vi "Test - Draw Teapot.vi"() -> ()   [LabVIEW 2022 SP3, in "Raster.lvlib"] (continued)
"y"=79.69716, "z"=0.98665166}, "UV"={"u"=0.0, "v"=0.0}, "Colour"=12517256}, "Alpha"=0.0, "Alpha Blending Enabled"=FALSE, "Colour"=131841}, {"Vertex 1"={"Position"={"x"=284.21167, "y"=415.62677, "z"=0.9870124}, "UV"={"u"=0.0, "v"=0.0}, "Colour"=12517256}, "Vertex 2"={"Position"={"x"=286.22012, "y"=416.7535, "z"=0.987065}, "UV"={"u"=0.0, "v"=0.0}, "Colour"=12517256}, "Vertex 3"={"Position"={"x"=308.5938, "y"=420.3274, "z"=0.9866676}, "UV"={"u"=0.0, "v"=0.0}, "Colour"=12517256}, "Alpha"=0.0, "Alpha Blending Enabled"=FALSE, "Colour"=11463293}, {"Vertex 1"={"Position"={"x"=457.236, "y"=406.36896, "z"=0.98676956}, "UV"={"u"=0.0, "v"=0.0}, "Colour"=12517256}, "Vertex 2"={"Position"={"x"=455.76038, "y"=411.28638, "z"=0.98685414}, "UV"={"u"=0.0, "v"=0.0}, "Colour"=12517256}, "Vertex 3"={"Position"={"x"=479.31567, "y"=409.0878, "z"=0.98711485}, "UV"={"u"=0.0, "v"=0.0}, "Colour"=12517256}, "Alpha"=0.0, "Alpha Blending Enabled"=FALSE, "Colour"=11595134}, {"Vertex 1"={"Position"={"x"=218.37251, "y"=136.46829, "z"=0.98655325}, "UV"={"u"=0.0, "v"=0.0}, "Colour"=12517256}, "Vertex 2"={"Position"={"x"=228.17778, "y"=127.85439, "z"=0.98674196}, "UV"={"u"=0.0, "v"=0.0}, "Colour"=12517256}, "Vertex 3"={"Position"={"x"=214.19673, "y"=136.68369, "z"=0.9874245}, "UV"={"u"=0.0, "v"=0.0}, "Colour"=12517256}, "Alpha"=0.0, "Alpha Blending Enabled"=FALSE, "Colour"=131841}, {"Vertex 1"={"Position"={"x"=523.7792, "y"=100.105064, "z"=0.9868028}, "UV"={"u"=0.0, "v"=0.0}, "Colour"=12517256}, "Vertex 2"={"Position"={"x"=527.92816, "y"=103.53234, "z"=0.986694}, "UV"={"u"=0.0, "v"=0.0}, "Colour"=12517256}, "Vertex 3"={"Position"={"x"=546.8862, "y"=111.29832, "z"=0.9872219}, "UV"={"u"=0.0, "v"=0.0}, "Colour"=12517256}, "Alpha"=0.0, "Alpha Blending Enabled"=FALSE, "Colour"=131841}, {"Vertex 1"={"Position"={"x"=429.0421, "y"=412.70264, "z"=0.9866862}, "UV"={"u"=0.0, "v"=0.0}, "Colour"=12517256}, "Vertex 2"={"Position"={"x"=426.95547, "y"=415.24643, "z"=0.98692787}, "UV"={"u"=0.0, "v"=0.0}, "Colour"=12517256}, "Vertex 3"={"Position"={"x"=451.80063, "y"=413.90112, "z"=0.987081}, "UV"={"u"=0.0, "v"=0.0}, "Colour"=12517256}, "Alpha"=0.0, "Alpha Blending Enabled"=FALSE, "Colour"=11726719}, {"Vertex 1"={"Position"={"x"=488.21274, "y"=84.37186, "z"=0.98678565}, "UV"={"u"=0.0, "v"=0.0}, "Colour"=12517256}, "Vertex 2"={"Position"={"x"=480.10406, "y"=86.833496, "z"=0.9870857}, "UV"={"u"=0.0, "v"=0.0}, "Colour"=12517256}, "Vertex 3"={"Position"={"x"=456.3261, "y"=82.49355, "z"=0.9868217}, "UV"={"u"=0.0, "v"=0.0}, "Colour"=12517256}, "Alpha"=0.0, "Alpha Blending Enabled"=FALSE, "Colour"=131841}, {"Vertex 1"={"Position"={"x"=513.7799, "y"=416.7535, "z"=0.987065}, "UV"={"u"=0.0, "v"=0.0}, "Colour"=12517256}, "Vertex 2"={"Position"={"x"=515.7883, "y"=415.62677, "z"=0.9870124}, "UV"={"u"=0.0, "v"=0.0}, "Colour"=12517256}, "Vertex 3"={"Position"={"x"=493.06995, "y"=419.2306, "z"=0.986606}, "UV"={"u"=0.0, "v"=0.0}, "Colour"=12517256}, "Alpha"=0.0, "Alpha Blending Enabled"=FALSE, "Colour"=11463293}, {"Vertex 1"={"Position"={"x"=344.2396, "y"=411.28638, "z"=0.98685414}, "UV"={"u"=0.0, "v"=0.0}, "Colour"=12517256}, "Vertex 2"={"Position"={"x"=342.764, "y"=406.36896, "z"=0.98676956}, "UV"={"u"=0.0, "v"=0.0}, "Colour"=12517256}, "Vertex 3"={"Position"={"x"=318.62802, "y"=404.213, "z"=0.98703873}, "UV"={"u"=0.0, "v"=0.0}, "Colour"=12517256}, "Alpha"=0.0, "Alpha Blending Enabled"=FALSE, "Colour"=11595134}, {"Vertex 1"={"Position"={"x"=277.7324, "y"=405.7855, "z"=0.9868424}, "UV"={"u"=0.0, "v"=0.0}, "Colour"=12517256}, "Vertex 2"={"Position"={"x"=269.55508, "y"=385.5468, "z"=0.98662794}, "UV"={"u"=0.0, "v"=0.0}, "Colour"=12517256}, "Vertex 3"={"Position"={"x"=250.34036, "y"=382.10144, "z"=0.98716855}, "UV"={"u"=0.0, "v"=0.0}, "Colour"=12517256}, "Alpha"=0.0, "Alpha Blending Enabled"=FALSE, "Colour"=9881963}, {"Vertex 1"={"Position"={"x"=451.80063, "y"=413.90112, "z"=0.987081}, "UV"={"u"=0.0, "v"=0.0}, "Colour"=12517256}, "Vertex 2"={"Position"={"x"=455.76038, "y"=411.28638, "z"=0.98685414}, "UV"={"u"=0.0, "v"=0.0}, "Colour"=12517256}, "Vertex 3"={"Position"={"x"=429.0421, "y"=412.70264, "z"=0.9866862}, "UV"={"u"=0.0, "v"=0.0}, "Colour"=12517256}, "Alpha"=0.0, "Alpha Blending Enabled"=FALSE, "Colour"=11726719}, {"Vertex 1"={"Position"={"x"=425.18686, "y"=85.50133, "z"=0.9871326}, "UV"={"u"=0.0, "v"=0.0}, "Colour"=12517256}, "Vertex 2"={"Position"={"x"=429.3405, "y"=79.69716, "z"=0.98665166}, "UV"={"u"=0.0, "v"=0.0}, "Colour"=12517256}, "Vertex 3"={"Position"={"x"=456.3261, "y"=82.49355, "z"=0.9868217}, "UV"={"u"=0.0, "v"=0.0}, "Colour"=12517256}, "Alpha"=0.0, "Alpha Blending Enabled"=FALSE, "Colour"=131841}, {"Vertex 1"={"Position"={"x"=571.8222, "y"=127.85439, "z"=0.98674196}, "UV"={"u"=0.0, "v"=0.0}, "Colour"=12517256}, "Vertex 2"={"Position"={"x"=581.62744, "y"=136.46829, "z"=0.98655325}, "UV"={"u"=0.0, "v"=0.0}, "Colour"=12517256}, "Vertex 3"={"Position"={"x"=595.8332, "y"=145.30861, "z"=0.9872829}, "UV"={"u"=0.0, "v"=0.0}, "Colour"=12517256}, "Alpha"=0.0, "Alpha Blending Enabled"=FALSE, "Colour"=131841}, {"Vertex 1"={"Position"={"x"=282.04407, "y"=413.45215, "z"=0.9869555}, "UV"={"u"=0.0, "v"=0.0}, "Colour"=12517256}, "Vertex 2"={"Position"={"x"=284.21167, "y"=415.62677, "z"=0.9870124}, "UV"={"u"=0.0, "v"=0.0}, "Colour"=12517256}, "Vertex 3"={"Position"={"x"=306.93005, "y"=419.2306, "z"=0.986606}, "UV"={"u"=0.0, "v"=0.0}, "Colour"=12517256}, "Alpha"=0.0, "Alpha Blending Enabled"=FALSE, "Colour"=11594878}, {"Vertex 1"={"Position"={"x"=549.6596, "y"=382.10144, "z"=0.98716855}, "UV"={"u"=0.0, "v"=0.0}, "Colour"=12517256}, "Vertex 2"={"Position"={"x"=558.7478, "y"=361.91916, "z"=0.9869936}, "UV"={"u"=0.0, "v"=0.0}, "Colour"=12517256}, "Vertex 3"={"Position"={"x"=538.7197, "y"=364.68237, "z"=0.986411}, "UV"={"u"=0.0, "v"=0.0}, "Colour"=12517256}, "Alpha"=0.0, "Alpha Blending Enabled"=FALSE, "Colour"=9816171}, {"Vertex 1"={"Position"={"x"=613.1543, "y"=168.46658, "z"=0.9870382}, "UV"={"u"=0.0, "v"=0.0}, "Colour"=12517256}, "Vertex 2"={"Position"={"x"=605.2505, "y"=155.83162, "z"=0.98714983}, "UV"={"u"=0.0, "v"=0.0}, "Colour"=12517256}, "Vertex 3"={"Position"={"x"=590.8862, "y"=147.17273, "z"=0.98637503}, "UV"={"u"=0.0, "v"=0.0}, "Colour"=12517256}, "Alpha"=0.0, "Alpha Blending Enabled"=FALSE, "Colour"=790537}, {"Vertex 1"={"Position"={"x"=188.08968, "y"=258.6834, "z"=0.9870558}, "UV"={"u"=0.0, "v"=0.0}, "Colour"=12517256}, "Vertex 2"={"Position"={"x"=194.1895, "y"=278.80545, "z"=0.98714197}, "UV"={"u"=0.0, "v"=0.0}, "Colour"=12517256}, "Vertex 3"={"Position"={"x"=208.56157, "y"=277.5288, "z"=0.9863644}, "UV"={"u"=0.0, "v"=0.0}, "Colour"=12517256}, "Alpha"=0.0, "Alpha Blending Enabled"=FALSE, "Colour"=8037207}, {"Vertex 1"={"Position"={"x"=562.28735, "y"=121.01229, "z"=0.9869255}, "UV"={"u"=0.0, "v"=0.0}, "Colour"=12517256}, "Vertex 2"={"Position"={"x"=553.7546, "y"=115.60594, "z"=0.98708975}, "UV"={"u"=0.0, "v"=0.0}, "Colour"=12517256}, "Vertex 3"={"Position"={"x"=534.1681, "y"=107.647095, "z"=0.9865303}, "UV"={"u"=0.0, "v"=0.0}, "Colour"=12517256}, "Alpha"=0.0, "Alpha Blending Enabled"=FALSE, "Colour"=131841}, {"Vertex 1"={"Position"={"x"=306.38147, "y"=83.88072, "z"=0.98658574}, "UV"={"u"=0.0, "v"=0.0}, "Colour"=12517256}, "Vertex 2"={"Position"={"x"=311.7873, "y"=84.37186, "z"=0.98678565}, "UV"={"u"=0.0, "v"=0.0}, "Colour"=12517256}, "Vertex 3"={"Position"={"x"=290.0812, "y"=90.55896, "z"=0.9871663}, "UV"={"u"=0.0, "v"=0.0}, "Colour"=12517256}, "Alpha"=0.0, "Alpha Blending Enabled"=FALSE, "Colour"=131841}, {"Vertex 1"={"Position"={"x"=584.2917, "y"=298.96686, "z"=0.98650193}, "UV"={"u"=0.0, "v"=0.0}, "Colour"=12517256}, "Vertex 2"={"Position"={"x"=576.293, "y"=320.26297, "z"=0.98665595}, "UV"={"u"=0.0, "v"=0.0}, "Colour"=12517256}, "Vertex 3"={"Position"={"x"=590.3839, "y"=319.19806, "z"=0.9873598}, "UV"={"u"=0.0, "v"=0.0}, "Colour"=12517256}, "Alpha"=0.0, "Alpha Blending Enabled"=FALSE, "Colour"=8564573}, {"Vertex 1"={"Position"={"x"=515.7883, "y"=415.62677, "z"=0.9870124}, "UV"={"u"=0.0, "v"=0.0}, "Colour"=12517256}, "Vertex 2"={"Position"={"x"=517.956, "y"=413.45215, "z"=0.9869555}, "UV"={"u"=0.0, "v"=0.0}, "Colour"=12517256}, "Vertex 3"={"Position"={"x"=494.86752, "y"=417.05643, "z"=0.9865395}, "UV"={"u"=0.0, "v"=0.0}, "Colour"=12517256}, "Alpha"=0.0, "Alpha Blending Enabled"=FALSE, "Colour"=11594878}, {"Vertex 1"={"Position"={"x"=491.4062, "y"=420.3274, "z"=0.9866676}, "UV"={"u"=0.0, "v"=0.0}, "Colour"=12517256}, "Vertex 2"={"Position"={"x"=489.97534, "y"=420.3969, "z"=0.9867205}, "UV"={"u"=0.0, "v"=0.0}, "Colour"=12517256}, "Vertex 3"={"Position"={"x"=512.05084, "y"=416.87537, "z"=0.9871104}, "UV"={"u"=0.0, "v"=0.0}, "Colour"=12517256}, "Alpha"=0.0, "Alpha Blending Enabled"=FALSE, "Colour"=10343280}, {"Vertex 1"={"Position"={"x"=370.9579, "y"=412.70264, "z"=0.9866862}, "UV"={"u"=0.0, "v"=0.0}, "Colour"=12517256}, "Vertex 2"={"Position"={"x"=373.04453, "y"=415.24643, "z"=0.98692787}, "UV"={"u"=0.0, "v"=0.0}, "Colour"=12517256}, "Vertex 3"={"Position"={"x"=400.0, "y"=415.71765, "z"=0.98687416}, "UV"={"u"=0.0, "v"=0.0}, "Colour"=12517256}, "Alpha"=0.0, "Alpha Blending Enabled"=FALSE, "Colour"=11792768}, {"Vertex 1"={"Position"={"x"=520.2092, "y"=91.74848, "z"=0.9868964}, "UV"={"u"=0.0, "v"=0.0}, "Colour"=12517256}, "Vertex 2"={"Position"={"x"=516.44995, "y"=90.450294, "z"=0.986995}, "UV"={"u"=0.0, "v"=0.0}, "Colour"=12517256}, "Vertex 3"={"Position"={"x"=493.61853, "y"=83.88072, "z"=0.98658574}, "UV"={"u"=0.0, "v"=0.0}, "Colour"=12517256}, "Alpha"=0.0, "Alpha Blending Enabled"=FALSE, "Colour"=131841}, {"Vertex 1"={"Position"={"x"=373.04453, "y"=415.24643, "z"=0.98692787}, "UV"={"u"=0.0, "v"=0.0}, "Colour"=12517256}, "Vertex 2"={"Position"={"x"=370.9579, "y"=412.70264, "z"=0.9866862}, "UV"={"u"=0.0, "v"=0.0}, "Colour"=12517256}, "Vertex 3"={"Position"={"x"=344.2396, "y"=411.28638, "z"=0.98685414}, "UV"={"u"=0.0, "v"=0.0}, "Colour"=12517256}, "Alpha"=0.0, "Alpha Blending Enabled"=FALSE, "Colour"=11726719}, {"Vertex 1"={"Position"={"x"=310.02466, "y"=420.3969, "z"=0.9867205}, "UV"={"u"=0.0, "v"=0.0}, "Colour"=12517256}, "Vertex 2"={"Position"={"x"=308.5938, "y"=420.3274, "z"=0.9866676}, "UV"={"u"=0.0, "v"=0.0}, "Colour"=12517256}, "Vertex 3"={"Position"={"x"=286.22012, "y"=416.7535, "z"=0.987065}, "UV"={"u"=0.0, "v"=0.0}, "Colour"=12517256}, "Alpha"=0.0, "Alpha Blending Enabled"=FALSE, "Colour"=10343280}, {"Vertex 1"={"Position"={"x"=265.8319, "y"=107.647095, "z"=0.9865303}, "UV"={"u"=0.0, "v"=0.0}, "Colour"=12517256}, "Vertex 2"={"Position"={"x"=272.07184, "y"=103.53234, "z"=0.986694}, "UV"={"u"=0.0, "v"=0.0}, "Colour"=12517256}, "Vertex 3"={"Position"={"x"=253.11374, "y"=111.29832, "z"=0.9872219}, "UV"={"u"=0.0, "v"=0.0}, "Colour"=12517256}, "Alpha"=0.0, "Alpha Blending Enabled"=FALSE, "Colour"=131841}, {"Vertex 1"={"Position"={"x"=605.8105, "y"=278.80545, "z"=0.98714197}, "UV"={"u"=0.0, "v"=0.0}, "Colour"=12517256}, "Vertex 2"={"Position"={"x"=611.91034, "y"=258.6834, "z"=0.9870558}, "UV"={"u"=0.0, "v"=0.0}, "Colour"=12517256}, "Vertex 3"={"Position"={"x"=597.4648, "y"=256.11636, "z"=0.98624843}, "UV"={"u"=0.0, "v"=0.0}, "Colour"=12517256}, "Alpha"=0.0, "Alpha Blending Enabled"=FALSE, "Colour"=8037207}, {"Vertex 1"={"Position"={"x"=400.0, "y"=413.19934, "z"=0.98662734}, "UV"={"u"=0.0, "v"=0.0}, "Colour"=12517256}, "Vertex 2"={"Position"={"x"=400.0, "y"=415.71765, "z"=0.98687416}, "UV"={"u"=0.0, "v"=0.0}, "Colour"=12517256}, "Vertex 3"={"Position"={"x"=426.95547, "y"=415.24643, "z"=0.98692787}, "UV"={"u"=0.0, "v"=0.0}, "Colour"=12517256}, "Alpha"=0.0, "Alpha Blending Enabled"=FALSE, "Colour"=11792768}, {"Vertex 1"={"Position"={"x"=194.7495, "y"=155.83162, "z"=0.98714983}, "UV"={"u"=0.0, "v"=0.0}, "Colour"=12517256}, "Vertex 2"={"Position"={"x"=186.84569, "y"=168.46658, "z"=0.9870382}, "UV"={"u"=0.0, "v"=0.0}, "Colour"=12517256}, "Vertex 3"={"Position"={"x"=201.30348, "y"=160.24332, "z"=0.9862247}, "UV"={"u"=0.0, "v"=0.0}, "Colour"=12517256}, "Alpha"=0.0, "Alpha Blending Enabled"=FALSE, "Colour"=790537}, {"Vertex 1"={"Position"={"x"=223.70695, "y"=320.26297, "z"=0.98665595}, "UV"={"u"=0.0, "v"=0.0}, "Colour"=12517256}, "Vertex 2"={"Position"={"x"=215.7083, "y"=298.96686, "z"=0.98650193}, "UV"={"u"=0.0, "v"=0.0}, "Colour"=12517256}, "Vertex 3"={"Position"={"x"=201.45174, "y"=299.0235, "z"=0.9872445}, "UV"={"u"=0.0, "v"=0.0}, "Colour"=12517256}, "Alpha"=0.0, "Alpha Blending Enabled"=FALSE, "Colour"=8564573}, {"Vertex 1"={"Position"={"x"=337.8442, "y"=79.5276, "z"=0.98648775}, "UV"={"u"=0.0, "v"=0.0}, "Colour"=12517256}, "Vertex 2"={"Position"={"x"=343.6739, "y"=82.49355, "z"=0.9868217}, "UV"={"u"=0.0, "v"=0.0}, "Colour"=12517256}, "Vertex 3"={"Position"={"x"=319.8959, "y"=86.833496, "z"=0.9870857}, "UV"={"u"=0.0, "v"=0.0}, "Colour"=12517256}, "Alpha"=0.0, "Alpha Blending Enabled"=FALSE, "Colour"=131841}, {"Vertex 1"={"Position"={"x"=279.84146, "y"=410.18558, "z"=0.9868977}, "UV"={"u"=0.0, "v"=0.0}, "Colour"=12517256}, "Vertex 2"={"Position"={"x"=282.04407, "y"=413.45215, "z"=0.9869555}, "UV"={"u"=0.0, "v"=0.0}, "Colour"=12517256}, "Vertex 3"={"Position"={"x"=305.13248, "y"=417.05643, "z"=0.9865395}, "UV"={"u"=0.0, "v"=0.0}, "Colour"=12517256}, "Alpha"=0.0, "Alpha Blending Enabled"=FALSE, "Colour"=11331451}, {"Vertex 1"={"Position"={"x"=374.81314, "y"=85.50133, "z"=0.9871326}, "UV"={"u"=0.0, "v"=0.0}, "Colour"=12517256}, "Vertex 2"={"Position"={"x"=370.6595, "y"=79.69716, "z"=0.98665166}, "UV"={"u"=0.0, "v"=0.0}, "Colour"=12517256}, "Vertex 3"={"Position"={"x"=400.0, "y"=78.71635, "z"=0.986592}, "UV"={"u"=0.0, "v"=0.0}, "Colour"=12517256}, "Alpha"=0.0, "Alpha Blending Enabled"=FALSE, "Colour"=131841}, {"Vertex 1"={"Position"={"x"=488.21274, "y"=84.37186, "z"=0.98678565}, "UV"={"u"=0.0, "v"=0.0}, "Colour"=12517256}, "Vertex 2"={"Position"={"x"=493.61853, "y"=83.88072, "z"=0.98658574}, "UV"={"u"=0.0, "v"=0.0}, "Colour"=12517256}, "Vertex 3"={"Position"={"x"=516.44995, "y"=90.450294, "z"=0.986995}, "UV"={"u"=0.0, "v"=0.0}, "Colour"=12517256}, "Alpha"=0.0, "Alpha Blending Enabled"=FALSE, "Colour"=131841}, {"Vertex 1"={"Position"={"x"=283.55002, "y"=90.450294, "z"=0.986995}, "UV"={"u"=0.0, "v"=0.0}, "Colour"=12517256}, "Vertex 2"={"Position"={"x"=279.79077, "y"=91.74848, "z"=0.9868964}, "UV"={"u"=0.0, "v"=0.0}, "Colour"=12517256}, "Vertex 3"={"Position"={"x"=303.26147, "y"=85.00194, "z"=0.9864703}, "UV"={"u"=0.0, "v"=0.0}, "Colour"=12517256}, "Alpha"=0.0, "Alpha Blending Enabled"=FALSE, "Colour"=131841}, {"Vertex 1"={"Position"={"x"=319.8959, "y"=86.833496, "z"=0.9870857}, "UV"={"u"=0.0, "v"=0.0}, "Colour"=12517256}, "Vertex 2"={"Position"={"x"=311.7873, "y"=84.37186, "z"=0.98678565}, "UV"={"u"=0.0, "v"=0.0}, "Colour"=12517256}, "Vertex 3"={"Position"={"x"=337.8442, "y"=79.5276, "z"=0.98648775}, "UV"={"u"=0.0, "v"=0.0}, "Colour"=12517256}, "Alpha"=0.0, "Alpha Blending Enabled"=FALSE, "Colour"=131841}, {"Vertex 1"={"Position"={"x"=246.24544, "y"=115.60594, "z"=0.98708975}, "UV"={"u"=0.0, "v"=0.0}, "Colour"=12517256}, "Vertex 2"={"Position"={"x"=237.71262, "y"=121.01229, "z"=0.9869255}, "UV"={"u"=0.0, "v"=0.0}, "Colour"=12517256}, "Vertex 3"={"Position"={"x"=258.046, "y"=112.83853, "z"=0.98632616}, "UV"={"u"=0.0, "v"=0.0}, "Colour"=12517256}, "Alpha"=0.0, "Alpha Blending Enabled"=FALSE, "Colour"=131841}, {"Vertex 1"={"Position"={"x"=493.06995, "y"=419.2306, "z"=0.986606}, "UV"={"u"=0.0, "v"=0.0}, "Colour"=12517256}, "Vertex 2"={"Position"={"x"=491.4062, "y"=420.3274, "z"=0.9866676}, "UV"={"u"=0.0, "v"=0.0}, "Colour"=12517256}, "Vertex 3"={"Position"={"x"=513.7799, "y"=416.7535, "z"=0.987065}, "UV"={"u"=0.0, "v"=0.0}, "Colour"=12517256}, "Alpha"=0.0, "Alpha Blending Enabled"=FALSE, "Colour"=11463293}, {"Vertex 1"={"Position"={"x"=400.0, "y"=84.68199, "z"=0.98708326}, "UV"={"u"=0.0, "v"=0.0}, "Colour"=12517256}, "Vertex 2"={"Position"={"x"=400.0, "y"=78.71635, "z"=0.986592}, "UV"={"u"=0.0, "v"=0.0}, "Colour"=12517256}, "Vertex 3"={"Position"={"x"=429.3405, "y"=79.69716, "z"=0.98665166}, "UV"={"u"=0.0, "v"=0.0}, "Colour"=12517256}, "Alpha"=0.0, "Alpha Blending Enabled"=FALSE, "Colour"=131841}, {"Vertex 1"={"Position"={"x"=517.956, "y"=413.45215, "z"=0.9869555}, "UV"={"u"=0.0, "v"=0.0}, "Colour"=12517256}, "Vertex 2"={"Position"={"x"=520.1585, "y"=410.18558, "z"=0.9868977}, "UV"={"u"=0.0, "v"=0.0}, "Colour"=12517256}, "Vertex 3"={"Position"={"x"=496.69638, "y"=413.75363, "z"=0.9864719}, "UV"={"u"=0.0, "v"=0.0}, "Colour"=12517256}, "Alpha"=0.0, "Alpha Blending Enabled"=FALSE, "Colour"=11331451}, {"Vertex 1"={"Position"={"x"=527.92816, "y"=103.53234, "z"=0.986694}, "UV"={"u"=0.0, "v"=0.0}, "Colour"=12517256}, "Vertex 2"={"Position"={"x"=534.1681, "y"=107.647095, "z"=0.9865303}, "UV"={"u"=0.0, "v"=0.0}, "Colour"=12517256}, "Vertex 3"={"Position"={"x"=553.7546, "y"=115.60594, "z"=0.98708975}, "UV"={"u"=0.0, "v"=0.0}, "Colour"=12517256}, "Alpha"=0.0, "Alpha Blending Enabled"=FALSE, "Colour"=131841}, {"Vertex 1"={"Position"={"x"=342.764, "y"=406.36896, "z"=0.98676956}, "UV"={"u"=0.0, "v"=0.0}, "Colour"=12517256}, "Vertex 2"={"Position"={"x"=344.2396, "y"=411.28638, "z"=0.98685414}, "UV"={"u"=0.0, "v"=0.0}, "Colour"=12517256}, "Vertex 3"={"Position"={"x"=370.9579, "y"=412.70264, "z"=0.9866862}, "UV"={"u"=0.0, "v"=0.0}, "Colour"=12517256}, "Alpha"=0.0, "Alpha Blending Enabled"=FALSE, "Colour"=11990146}, {"Vertex 1"={"Position"={"x"=183.4162, "y"=238.81894, "z"=0.98698974}, "UV"={"u"=0.0, "v"=0.0}, "Colour"=12517256}, "Vertex 2"={"Position"={"x"=188.08968, "y"=258.6834, "z"=0.9870558}, "UV"={"u"=0.0, "v"=0.0}, "Colour"=12517256}, "Vertex 3"={"Position"={"x"=202.53506, "y"=256.11636, "z"=0.98624843}, "UV"={"u"=0.0, "v"=0.0}, "Colour"=12517256}, "Alpha"=0.0, "Alpha Blending Enabled"=FALSE, "Colour"=7576146}, {"Vertex 1"={"Position"={"x"=308.5938, "y"=420.3274, "z"=0.9866676}, "UV"={"u"=0.0, "v"=0.0}, "Colour"=12517256}, "Vertex 2"={"Position"={"x"=306.93005, "y"=419.2306, "z"=0.986606}, "UV"={"u"=0.0, "v"=0.0}, "Colour"=12517256}, "Vertex 3"={"Position"={"x"=284.21167, "y"=415.62677, "z"=0.9870124}, "UV"={"u"=0.0, "v"=0.0}, "Colour"=12517256}, "Alpha"=0.0, "Alpha Blending Enabled"=FALSE, "Colour"=11463293}, {"Vertex 1"={"Position"={"x"=426.95547, "y"=415.24643, "z"=0.98692787}, "UV"={"u"=0.0, "v"=0.0}, "Colour"=12517256}, "Vertex 2"={"Position"={"x"=429.0421, "y"=412.70264, "z"=0.9866862}, "UV"={"u"=0.0, "v"=0.0}, "Colour"=12517256}, "Vertex 3"={"Position"={"x"=400.0, "y"=413.19934, "z"=0.98662734}, "UV"={"u"=0.0, "v"=0.0}, "Colour"=12517256}, "Alpha"=0.0, "Alpha Blending Enabled"=FALSE, "Colour"=11792768}, {"Vertex 1"={"Position"={"x"=232.30115, "y"=341.28168, "z"=0.98682135}, "UV"={"u"=0.0, "v"=0.0}, "Colour"=12517256}, "Vertex 2"={"Position"={"x"=241.25218, "y"=361.91916, "z"=0.9869936}, "UV"={"u"=0.0, "v"=0.0}, "Colour"=12517256}, "Vertex 3"={"Position"={"x"=261.2803, "y"=364.68237, "z"=0.986411}, "UV"={"u"=0.0, "v"=0.0}, "Colour"=12517256}, "Alpha"=0.0, "Alpha Blending Enabled"=FALSE, "Colour"=9750378}, {"Vertex 1"={"Position"={"x"=618.5962, "y"=183.36784, "z"=0.98696136}, "UV"={"u"=0.0, "v"=0.0}, "Colour"=12517256}, "Vertex 2"={"Position"={"x"=613.1543, "y"=168.46658, "z"=0.9870382}, "UV"={"u"=0.0, "v"=0.0}, "Colour"=12517256}, "Vertex 3"={"Position"={"x"=598.69653, "y"=160.24332, "z"=0.9862247}, "UV"={"u"=0.0, "v"=0.0}, "Colour"=12517256}, "Alpha"=0.0, "Alpha Blending Enabled"=FALSE, "Colour"=2701085}, {"Vertex 1"={"Position"={"x"=455.76038, "y"=411.28638, "z"=0.98685414}, "UV"={"u"=0.0, "v"=0.0}, "Colour"=12517256}, "Vertex 2"={"Position"={"x"=457.236, "y"=406.36896, "z"=0.98676956}, "UV"={"u"=0.0, "v"=0.0}, "Colour"=12517256}, "Vertex 3"={"Position"={"x"=429.82074, "y"=407.75894, "z"=0.986596}, "UV"={"u"=0.0, "v"=0.0}, "Colour"=12517256}, "Alpha"=0.0, "Alpha Blending Enabled"=FALSE, "Colour"=11990146}, {"Vertex 1"={"Position"={"x"=521.88837, "y"=94.06487, "z"=0.98685235}, "UV"={"u"=0.0, "v"=0.0}, "Colour"=12517256}, "Vertex 2"={"Position"={"x"=520.2092, "y"=91.74848, "z"=0.9868964}, "UV"={"u"=0.0, "v"=0.0}, "Colour"=12517256}, "Vertex 3"={"Position"={"x"=496.73853, "y"=85.00194, "z"=0.9864703}, "UV"={"u"=0.0, "v"=0.0}, "Colour"=12517256}, "Alpha"=0.0, "Alpha Blending Enabled"=FALSE, "Colour"=988171}, {"Vertex 1"={"Position"={"x"=277.7324, "y"=405.7855, "z"=0.9868424}, "UV"={"u"=0.0, "v"=0.0}, "Colour"=12517256}, "Vertex 2"={"Position"={"x"=279.84146, "y"=410.18558, "z"=0.9868977}, "UV"={"u"=0.0, "v"=0.0}, "Colour"=12517256}, "Vertex 3"={"Position"={"x"=303.30362, "y"=413.75363, "z"=0.9864719}, "UV"={"u"=0.0, "v"=0.0}, "Colour"=12517256}, "Alpha"=0.0, "Alpha Blending Enabled"=FALSE, "Colour"=10870390}, {"Vertex 1"={"Position"={"x"=209.11378, "y"=147.17273, "z"=0.98637503}, "UV"={"u"=0.0, "v"=0.0}, "Colour"=12517256}, "Vertex 2"={"Position"={"x"=218.37251, "y"=136.46829, "z"=0.98655325}, "UV"={"u"=0.0, "v"=0.0}, "Colour"=12517256}, "Vertex 3"={"Position"={"x"=204.1668, "y"=145.30861, "z"=0.9872829}, "UV"={"u"=0.0, "v"=0.0}, "Colour"=12517256}, "Alpha"=0.0, "Alpha Blending Enabled"=FALSE, "Colour"=131841}, {"Vertex 1"={"Position"={"x"=538.7197, "y"=364.68237, "z"=0.986411}, "UV"={"u"=0.0, "v"=0.0}, "Colour"=12517256}, "Vertex 2"={"Position"={"x"=530.4449, "y"=385.5468, "z"=0.98662794}, "UV"={"u"=0.0, "v"=0.0}, "Colour"=12517256}, "Vertex 3"={"Position"={"x"=549.6596, "y"=382.10144, "z"=0.98716855}, "UV"={"u"=0.0, "v"=0.0}, "Colour"=12517256}, "Alpha"=0.0, "Alpha Blending Enabled"=FALSE, "Colour"=9816171}, {"Vertex 1"={"Position"={"x"=611.91034, "y"=258.6834, "z"=0.9870558}, "UV"={"u"=0.0, "v"=0.0}, "Colour"=12517256}, "Vertex 2"={"Position"={"x"=616.5838, "y"=238.81894, "z"=0.98698974}, "UV"={"u"=0.0, "v"=0.0}, "Colour"=12517256}, "Vertex 3"={"Position"={"x"=602.0967, "y"=234.92854, "z"=0.98615927}, "UV"={"u"=0.0, "v"=0.0}, "Colour"=12517256}, "Alpha"=0.0, "Alpha Blending Enabled"=FALSE, "Colour"=7576146}, {"Vertex 1"={"Position"={"x"=400.0, "y"=415.71765, "z"=0.98687416}, "UV"={"u"=0.0, "v"=0.0}, "Colour"=12517256}, "Vertex 2"={"Position"={"x"=400.0, "y"=413.19934, "z"=0.98662734}, "UV"={"u"=0.0, "v"=0.0}, "Colour"=12517256}, "Vertex 3"={"Position"={"x"=370.9579, "y"=412.70264, "z"=0.9866862}, "UV"={"u"=0.0, "v"=0.0}, "Colour"=12517256}, "Alpha"=0.0, "Alpha Blending Enabled"=FALSE, "Colour"=11792768}, {"Vertex 1"={"Position"={"x"=279.79077, "y"=91.74848, "z"=0.9868964}, "UV"={"u"=0.0, "v"=0.0}, "Colour"=12517256}, "Vertex 2"={"Position"={"x"=278.11163, "y"=94.06487, "z"=0.98685235}, "UV"={"u"=0.0, "v"=0.0}, "Colour"=12517256}, "Vertex 3"={"Position"={"x"=301.8657, "y"=87.29713, "z"=0.98641866}, "UV"={"u"=0.0, "v"=0.0}, "Colour"=12517256}, "Alpha"=0.0, "Alpha Blending Enabled"=FALSE, "Colour"=988171}, {"Vertex 1"={"Position"={"x"=494.86752, "y"=417.05643, "z"=0.9865395}, "UV"={"u"=0.0, "v"=0.0}, "Colour"=12517256}, "Vertex 2"={"Position"={"x"=493.06995, "y"=419.2306, "z"=0.986606}, "UV"={"u"=0.0, "v"=0.0}, "Colour"=12517256}, "Vertex 3"={"Position"={"x"=515.7883, "y"=415.62677, "z"=0.9870124}, "UV"={"u"=0.0, "v"=0.0}, "Colour"=12517256}, "Alpha"=0.0, "Alpha Blending Enabled"=FALSE, "Colour"=11594878}, {"Vertex 1"={"Position"={"x"=520.1585, "y"=410.18558, "z"=0.9868977}, "UV"={"u"=0.0, "v"=0.0}, "Colour"=12517256}, "Vertex 2"={"Position"={"x"=522.26764, "y"=405.7855, "z"=0.9868424}, "UV"={"u"=0.0, "v"=0.0}, "Colour"=12517256}, "Vertex 3"={"Position"={"x"=498.44965, "y"=409.27316, "z"=0.986407}, "UV"={"u"=0.0, "v"=0.0}, "Colour"=12517256}, "Alpha"=0.0, "Alpha Blending Enabled"=FALSE, "Colour"=10870390}, {"Vertex 1"={"Position"={"x"=429.82074, "y"=407.75894, "z"=0.986596}, "UV"={"u"=0.0, "v"=0.0}, "Colour"=12517256}, "Vertex 2"={"Position"={"x"=429.0421, "y"=412.70264, "z"=0.9866862}, "UV"={"u"=0.0, "v"=0.0}, "Colour"=12517256}, "Vertex 3"={"Position"={"x"=455.76038, "y"=411.28638, "z"=0.98685414}, "UV"={"u"=0.0, "v"=0.0}, "Colour"=12517256}, "Alpha"=0.0, "Alpha Blending Enabled"=FALSE, "Colour"=11990146}, {"Vertex 1"={"Position"={"x"=186.84569, "y"=168.46658, "z"=0.9870382}, "UV"={"u"=0.0, "v"=0.0}, "Colour"=12517256}, "Vertex 2"={"Position"={"x"=181.40381, "y"=183.36784, "z"=0.98696136}, "UV"={"u"=0.0, "v"=0.0}, "Colour"=12517256}, "Vertex 3"={"Position"={"x"=195.90497, "y"=175.87807, "z"=0.9861208}, "UV"={"u"=0.0, "v"=0.0}, "Colour"=12517256}, "Alpha"=0.0, "Alpha Blending Enabled"=FALSE, "Colour"=2701085}, {"Vertex 1"={"Position"={"x"=522.26764, "y"=96.98737, "z"=0.9868424}, "UV"={"u"=0.0, "v"=0.0}, "Colour"=12517256}, "Vertex 2"={"Position"={"x"=521.88837, "y"=94.06487, "z"=0.98685235}, "UV"={"u"=0.0, "v"=0.0}, "Colour"=12517256}, "Vertex 3"={"Position"={"x"=498.13428, "y"=87.29713, "z"=0.98641866}, "UV"={"u"=0.0, "v"=0.0}, "Colour"=12517256}, "Alpha"=0.0, "Alpha Blending Enabled"=FALSE, "Colour"=6061122}, {"Vertex 1"={"Position"={"x"=591.4384, "y"=277.5288, "z"=0.9863644}, "UV"={"u"=0.0, "v"=0.0}, "Colour"=12517256}, "Vertex 2"={"Position"={"x"=584.2917, "y"=298.96686, "z"=0.98650193}, "UV"={"u"=0.0, "v"=0.0}, "Colour"=12517256}, "Vertex 3"={"Position"={"x"=598.5483, "y"=299.0235, "z"=0.9872445}, "UV"={"u"=0.0, "v"=0.0}, "Colour"=12517256}, "Alpha"=0.0, "Alpha Blending Enabled"=FALSE, "Colour"=8366683}, {"Vertex 1"={"Position"={"x"=278.11163, "y"=94.06487, "z"=0.98685235}, "UV"={"u"=0.0, "v"=0.0}, "Colour"=12517256}, "Vertex 2"={"Position"={"x"=277.7324, "y"=96.98737, "z"=0.9868424}, "UV"={"u"=0.0, "v"=0.0}, "Colour"=12517256}, "Vertex 3"={"Position"={"x"=301.55032, "y"=90.294205, "z"=0.986407}, "UV"={"u"=0.0, "v"=0.0}, "Colour"=12517256}, "Alpha"=0.0, "Alpha Blending Enabled"=FALSE, "Colour"=6061122}, {"Vertex 1"={"Position"={"x"=306.93005, "y"=419.2306, "z"=0.986606}, "UV"={"u"=0.0, "v"=0.0}, "Colour"=12517256}, "Vertex 2"={"Position"={"x"=305.13248, "y"=417.05643, "z"=0.9865395}, "UV"={"u"=0.0, "v"=0.0}, "Colour"=12517256}, "Vertex 3"={"Position"={"x"=282.04407, "y"=413.45215, "z"=0.9869555}, "UV"={"u"=0.0, "v"=0.0}, "Colour"=12517256}, "Alpha"=0.0, "Alpha Blending Enabled"=FALSE, "Colour"=11594878}, {"Vertex 1"={"Position"={"x"=180.43036, "y"=219.3934, "z"=0.98694754}, "UV"={"u"=0.0, "v"=0.0}, "Colour"=12517256}, "Vertex 2"={"Position"={"x"=183.4162, "y"=238.81894, "z"=0.98698974}, "UV"={"u"=0.0, "v"=0.0}, "Colour"=12517256}, "Vertex 3"={"Position"={"x"=197.90335, "y"=234.92854, "z"=0.98615927}, "UV"={"u"=0.0, "v"=0.0}, "Colour"=12517256}, "Alpha"=0.0, "Alpha Blending Enabled"=FALSE, "Colour"=6983244}, {"Vertex 1"={"Position"={"x"=456.3261, "y"=82.49355, "z"=0.9868217}, "UV"={"u"=0.0, "v"=0.0}, "Colour"=12517256}, "Vertex 2"={"Position"={"x"=462.15582, "y"=79.5276, "z"=0.98648775}, "UV"={"u"=0.0, "v"=0.0}, "Colour"=12517256}, "Vertex 3"={"Position"={"x"=488.21274, "y"=84.37186, "z"=0.98678565}, "UV"={"u"=0.0, "v"=0.0}, "Colour"=12517256}, "Alpha"=0.0, "Alpha Blending Enabled"=FALSE, "Colour"=131841}, {"Vertex 1"={"Position"={"x"=581.62744, "y"=136.46829, "z"=0.98655325}, "UV"={"u"=0.0, "v"=0.0}, "Colour"=12517256}, "Vertex 2"={"Position"={"x"=590.8862, "y"=147.17273, "z"=0.98637503}, "UV"={"u"=0.0, "v"=0.0}, "Colour"=12517256}, "Vertex 3"={"Position"={"x"=605.2505, "y"=155.83162, "z"=0.98714983}, "UV"={"u"=0.0, "v"=0.0}, "Colour"=12517256}, "Alpha"=0.0, "Alpha Blending Enabled"=FALSE, "Colour"=131841}, {"Vertex 1"={"Position"={"x"=523.7792, "y"=100.105064, "z"=0.9868028}, "UV"={"u"=0.0, "v"=0.0}, "Colour"=12517256}, "Vertex 2"={"Position"={"x"=522.26764, "y"=96.98737, "z"=0.9868424}, "UV"={"u"=0.0, "v"=0.0}, "Colour"=12517256}, "Vertex 3"={"Position"={"x"=498.44965, "y"=90.294205, "z"=0.986407}, "UV"={"u"=0.0, "v"=0.0}, "Colour"=12517256}, "Alpha"=0.0, "Alpha Blending Enabled"=FALSE, "Colour"=2635293}, {"Vertex 1"={"Position"={"x"=370.9579, "y"=412.70264, "z"=0.9866862}, "UV"={"u"=0.0, "v"=0.0}, "Colour"=12517256}, "Vertex 2"={"Position"={"x"=370.17926, "y"=407.75894, "z"=0.986596}, "UV"={"u"=0.0, "v"=0.0}, "Colour"=12517256}, "Vertex 3"={"Position"={"x"=342.764, "y"=406.36896, "z"=0.98676956}, "UV"={"u"=0.0, "v"=0.0}, "Colour"=12517256}, "Alpha"=0.0, "Alpha Blending Enabled"=FALSE, "Colour"=11990146}, {"Vertex 1"={"Position"={"x"=303.26147, "y"=85.00194, "z"=0.9864703}, "UV"={"u"=0.0, "v"=0.0}, "Colour"=12517256}, "Vertex 2"={"Position"={"x"=306.38147, "y"=83.88072, "z"=0.98658574}, "UV"={"u"=0.0, "v"=0.0}, "Colour"=12517256}, "Vertex 3"={"Position"={"x"=283.55002, "y"=90.450294, "z"=0.986995}, "UV"={"u"=0.0, "v"=0.0}, "Colour"=12517256}, "Alpha"=0.0, "Alpha Blending Enabled"=FALSE, "Colour"=131841}, {"Vertex 1"={"Position"={"x"=616.5838, "y"=238.81894, "z"=0.98698974}, "UV"={"u"=0.0, "v"=0.0}, "Colour"=12517256}, "Vertex 2"={"Position"={"x"=619.56964, "y"=219.3934, "z"=0.98694754}, "UV"={"u"=0.0, "v"=0.0}, "Colour"=12517256}, "Vertex 3"={"Position"={"x"=605.0625, "y"=214.19258, "z"=0.9861022}, "UV"={"u"=0.0, "v"=0.0}, "Colour"=12517256}, "Alpha"=0.0, "Alpha Blending Enabled"=FALSE, "Colour"=6983244}, {"Vertex 1"={"Position"={"x"=269.55508, "y"=385.5468, "z"=0.98662794}, "UV"={"u"=0.0, "v"=0.0}, "Colour"=12517256}, "Vertex 2"={"Position"={"x"=261.2803, "y"=364.68237, "z"=0.986411}, "UV"={"u"=0.0, "v"=0.0}, "Colour"=12517256}, "Vertex 3"={"Position"={"x"=241.25218, "y"=361.91916, "z"=0.9869936}, "UV"={"u"=0.0, "v"=0.0}, "Colour"=12517256}, "Alpha"=0.0, "Alpha Blending Enabled"=FALSE, "Colour"=9816171}, {"Vertex 1"={"Position"={"x"=620.6173, "y"=200.60477, "z"=0.98693275}, "UV"={"u"=0.0, "v"=0.0}, "Colour"=12517256}, "Vertex 2"={"Position"={"x"=618.5962, "y"=183.36784, "z"=0.98696136}, "UV"={"u"=0.0, "v"=0.0}, "Colour"=12517256}, "Vertex 3"={"Position"={"x"=604.09503, "y"=175.87807, "z"=0.9861208}, "UV"={"u"=0.0, "v"=0.0}, "Colour"=12517256}, "Alpha"=0.0, "Alpha Blending Enabled"=FALSE, "Colour"=4743476}, {"Vertex 1"={"Position"={"x"=558.7478, "y"=361.91916, "z"=0.9869936}, "UV"={"u"=0.0, "v"=0.0}, "Colour"=12517256}, "Vertex 2"={"Position"={"x"=567.69885, "y"=341.28168, "z"=0.98682135}, "UV"={"u"=0.0, "v"=0.0}, "Colour"=12517256}, "Vertex 3"={"Position"={"x"=546.9111, "y"=343.2327, "z"=0.98619616}, "UV"={"u"=0.0, "v"=0.0}, "Colour"=12517256}, "Alpha"=0.0, "Alpha Blending Enabled"=FALSE, "Colour"=9750378}, {"Vertex 1"={"Position"={"x"=215.7083, "y"=298.96686, "z"=0.98650193}, "UV"={"u"=0.0, "v"=0.0}, "Colour"=12517256}, "Vertex 2"={"Position"={"x"=208.56157, "y"=277.5288, "z"=0.9863644}, "UV"={"u"=0.0, "v"=0.0}, "Colour"=12517256}, "Vertex 3"={"Position"={"x"=194.1895, "y"=278.80545, "z"=0.98714197}, "UV"={"u"=0.0, "v"=0.0}, "Colour"=12517256}, "Alpha"=0.0, "Alpha Blending Enabled"=FALSE, "Colour"=8366683}, {"Vertex 1"={"Position"={"x"=277.7324, "y"=96.98737, "z"=0.9868424}, "UV"={"u"=0.0, "v"=0.0}, "Colour"=12517256}, "Vertex 2"={"Position"={"x"=276.2208, "y"=100.105064, "z"=0.9868028}, "UV"={"u"=0.0, "v"=0.0}, "Colour"=12517256}, "Vertex 3"={"Position"={"x"=300.29266, "y"=93.43051, "z"=0.98636043}, "UV"={"u"=0.0, "v"=0.0}, "Colour"=12517256}, "Alpha"=0.0, "Alpha Blending Enabled"=FALSE, "Colour"=2635293}, {"Vertex 1"={"Position"={"x"=571.8222, "y"=127.85439, "z"=0.98674196}, "UV"={"u"=0.0, "v"=0.0}, "Colour"=12517256}, "Vertex 2"={"Position"={"x"=562.28735, "y"=121.01229, "z"=0.9869255}, "UV"={"u"=0.0, "v"=0.0}, "Colour"=12517256}, "Vertex 3"={"Position"={"x"=541.95404, "y"=112.83853, "z"=0.98632616}, "UV"={"u"=0.0, "v"=0.0}, "Colour"=12517256}, "Alpha"=0.0, "Alpha Blending Enabled"=FALSE, "Colour"=131841}, {"Vertex 1"={"Position"={"x"=179.3827, "y"=200.60477, "z"=0.98693275}, "UV"={"u"=0.0, "v"=0.0}, "Colour"=12517256}, "Vertex 2"={"Position"={"x"=180.43036, "y"=219.3934, "z"=0.98694754}, "UV"={"u"=0.0, "v"=0.0}, "Colour"=12517256}, "Vertex 3"={"Position"={"x"=194.93755, "y"=214.19258, "z"=0.9861022}, "UV"={"u"=0.0, "v"=0.0}, "Colour"=12517256}, "Alpha"=0.0, "Alpha Blending Enabled"=FALSE, "Colour"=6192963}, {"Vertex 1"={"Position"={"x"=181.40381, "y"=183.36784, "z"=0.98696136}, "UV"={"u"=0.0, "v"=0.0}, "Colour"=12517256}, "Vertex 2"={"Position"={"x"=179.3827, "y"=200.60477, "z"=0.98693275}, "UV"={"u"=0.0, "v"=0.0}, "Colour"=12517256}, "Vertex 3"={"Position"={"x"=193.89563, "y"=194.15904, "z"=0.98608214}, "UV"={"u"=0.0, "v"=0.0}, "Colour"=12517256}, "Alpha"=0.0, "Alpha Blending Enabled"=FALSE, "Colour"=4743476}, {"Vertex 1"={"Position"={"x"=496.69638, "y"=413.75363, "z"=0.9864719}, "UV"={"u"=0.0, "v"=0.0}, "Colour"=12517256}, "Vertex 2"={"Position"={"x"=494.86752, "y"=417.05643, "z"=0.9865395}, "UV"={"u"=0.0, "v"=0.0}, "Colour"=12517256}, "Vertex 3"={"Position"={"x"=517.956, "y"=413.45215, "z"=0.9869555}, "UV"={"u"=0.0, "v"=0.0}, "Colour"=12517256}, "Alpha"=0.0, "Alpha Blending Enabled"=FALSE, "Colour"=11331451}, {"Vertex 1"={"Position"={"x"=619.56964, "y"=219.3934, "z"=0.98694754}, "UV"={"u"=0.0, "v"=0.0}, "Colour"=12517256}, "Vertex 2"={"Position"={"x"=620.6173, "y"=200.60477, "z"=0.98693275}, "UV"={"u"=0.0, "v"=0.0}, "Colour"=12517256}, "Vertex 3"={"Position"={"x"=606.1044, "y"=194.15904, "z"=0.98608214}, "UV"={"u"=0.0, "v"=0.0}, "Colour"=12517256}, "Alpha"=0.0, "Alpha Blending Enabled"=FALSE, "Colour"=6192963}, {"Vertex 1"={"Position"={"x"=462.15582, "y"=79.5276, "z"=0.98648775}, "UV"={"u"=0.0, "v"=0.0}, "Colour"=12517256}, "Vertex 2"={"Position"={"x"=456.3261, "y"=82.49355, "z"=0.9868217}, "UV"={"u"=0.0, "v"=0.0}, "Colour"=12517256}, "Vertex 3"={"Position"={"x"=429.3405, "y"=79.69716, "z"=0.98665166}, "UV"={"u"=0.0, "v"=0.0}, "Colour"=12517256}, "Alpha"=0.0, "Alpha Blending Enabled"=FALSE, "Colour"=131841}, {"Vertex 1"={"Position"={"x"=493.61853, "y"=83.88072, "z"=0.98658574}, "UV"={"u"=0.0, "v"=0.0}, "Colour"=12517256}, "Vertex 2"={"Position"={"x"=496.73853, "y"=85.00194, "z"=0.9864703}, "UV"={"u"=0.0, "v"=0.0}, "Colour"=12517256}, "Vertex 3"={"Position"={"x"=520.2092, "y"=91.74848, "z"=0.9868964}, "UV"={"u"=0.0, "v"=0.0}, "Colour"=12517256}, "Alpha"=0.0, "Alpha Blending Enabled"=FALSE, "Colour"=131841}, {"Vertex 1"={"Position"={"x"=258.046, "y"=112.83853, "z"=0.98632616}, "UV"={"u"=0.0, "v"=0.0}, "Colour"=12517256}, "Vertex 2"={"Position"={"x"=265.8319, "y"=107.647095,
